vi "status.vi"(8 "error IO":errorcluster, 11 "enable":bool[](array[boolean])) -> (0 "error out":errorcluster, 2 "Actual Positions":i32[](array[numeric]), 3 "stopped?":bool[](array[boolean]))   [LabVIEW 2013, in "PicoMotor.lvclass"]
uses:
  PicoMotor.lvclass
  PicoMotor.lvclass/PicoMotor.ctl
  Globals.vi
panel:
  in  "PicoMotor.lvclass":refnum<class "PicoMotor.lvclass">
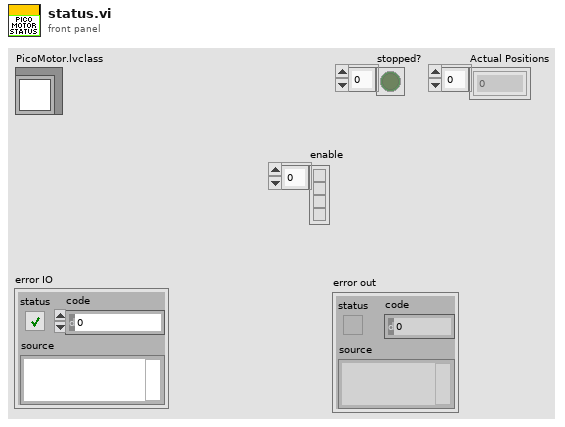
[diagram p1: front panel]
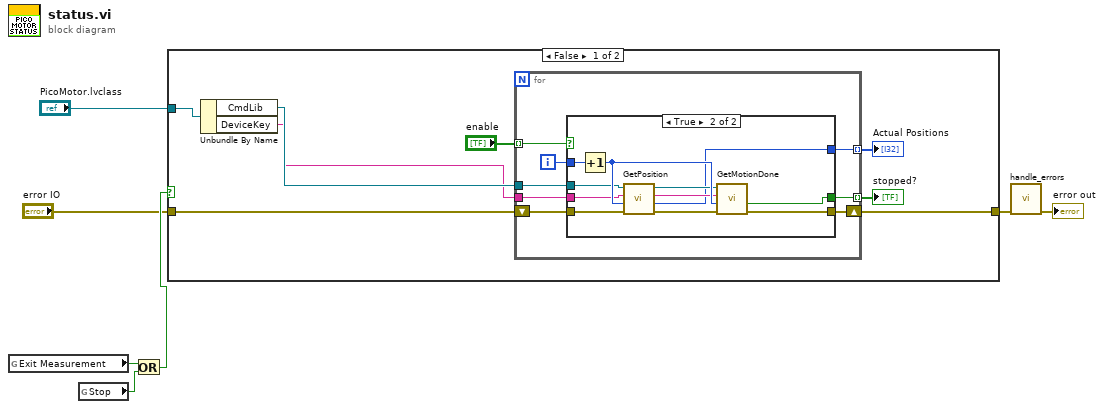
[diagram p0: block diagram]
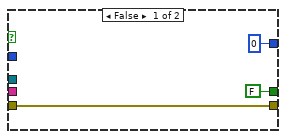
[diagram p2: hidden frame]
diagram:
  n1 = global read "Globals.vi" "Exit Measurement"() -> (w5:bool)
  n2 = global read "Globals.vi" "Stop"() -> (w4:bool)
  n3 = Or(x=w5, y=w4) -> (x .or. y?=w3:bool)
  n4 = case shown="False" w3 {
    tunnel: [w15 w38] -> w7
    tunnel: "error IO" -> [w8 w38]
    tunnel: "PicoMotor.lvclass" -> [w11 _]
    frame False {
      n5 = Unbundle By Name(w11) -> ("CmdLib"=w10:refnum<k24>, "DeviceKey"=w9:string)
      n6 = for {
        shift-right: [w19] -> w15
        shift-left: w8 -> [w22]
        tunnel: w9 -> [w21]
        tunnel: w10 -> [w20]
        tunnel: [w18] -> w14 mode=indexing
        tunnel: [w17] -> w13 mode=indexing
        tunnel: "enable" -> [w16] mode=indexing
        i -> [w23]
        n7 = case shown="True" w16 {
          tunnel: w23 -> [_ w37]
          tunnel: w22 -> [w26 w29]
          tunnel: w21 -> [_ w30]
          tunnel: w20 -> [_ w31]
          tunnel: [w26 w32] -> w19
          tunnel: [FALSE ("Is Motion Done") w28] -> w18
          tunnel: [0 ("Position") w27] -> w17
          frame False {
          }
          frame True {
            n8 = Increment(x=w37) -> (x+1=w35:i32)
            n9 = call "GetPosition.vi"("error in (no error)"=w29, "Motor"=w35, "DeviceKey In"=w30, "CmdLib In"=w31) -> ("error out"=w36:errorcluster, "Position"=w27:i32, "DeviceKey Out"=w33:string, "CmdLib Out"=w34:refnum<k24>)
            n10 = call "GetMotionDone.vi"("error in (no error)"=w36, "Motor"=w35, "DeviceKey In"=w33, "CmdLib In"=w34) -> ("error out"=w32:errorcluster, "Is Motion Done"=w28:bool)  [unwired: 2 out]
          }
        }
      }
      "stopped?" <- w14
      "Actual Positions" <- w13
    }
    frame True {
    }
  }
  n11 = call "handle_errors.vi"("error in (no error)"=w7) -> ("error out"=→"error out":errorcluster)  [unwired: 14 in]
